vi "FTW-ERR-UnknownMessage.vi"(8 "error in":errorcluster, 9 "Sender":string, 10 "Unknown Parameter":string) -> (0 "error out":errorcluster)   [LabVIEW 2013]
panel:
  # "Inputs"
  # "Outputs"
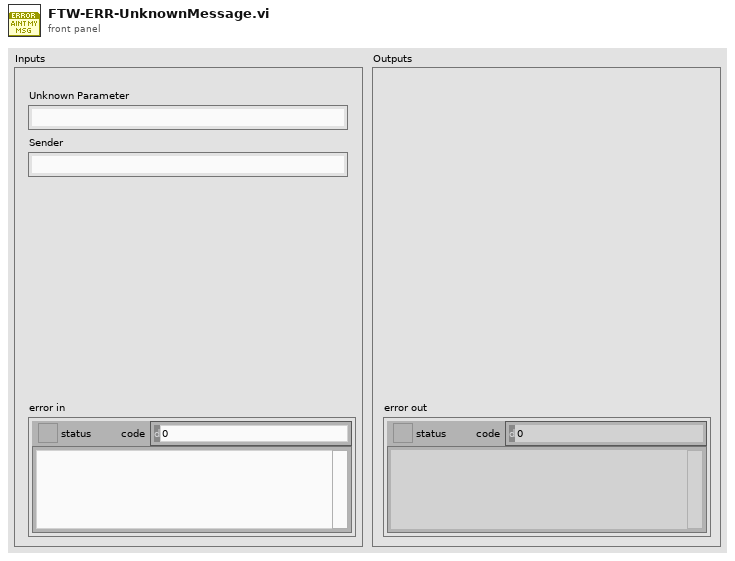
[diagram p1: front panel]
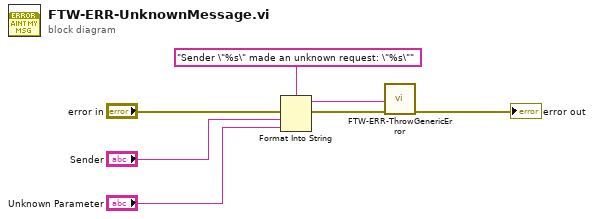
[diagram p0: block diagram]
diagram:
  n1 = Format Into String(format string="Sender \"%s\" made an unknown request: \"%s\"", error in="error in", "Sender", "Unknown Parameter") -> (resulting string=w4:string, error out=w5:errorcluster)  [unwired: 1 in]
  n2 = call "FTW-ERR-ThrowGenericError.vi"("Error Message"=w4, "error in"=w5) -> ("error out"=→"error out":errorcluster)  [unwired: 13 in]
